vi "Get Unique Test ID.vi"(1 "Basic DAQ Board in":refnum<class "Basic DAQ Design.lvclass">) -> (0 "id #":u32)   [LabVIEW 2023, in "Basic DAQ Design.lvclass"]
doc: "Get an identification number."
uses:
  Basic DAQ Design.lvclass
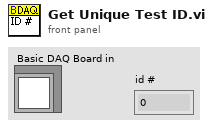
[diagram p1: front panel]
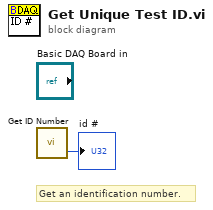
[diagram p0: block diagram]
diagram:
  # "Get an identification number."
  n1 = call "Get ID Number.vi"() -> ("id number"=→"id #":u32)  [unwired: 2 in]
